vi "Load Subsystem IO Attributes.vi"(8 "error in (no error)":errorcluster, 11 "Subsystem I/O Attributes File Path":path) -> (0 "error out":errorcluster, 3 "Subsystem I/O Attributes":T1[](array[typedef]))   [LabVIEW 2024]
doc: "Load subsystem I/O attributes from the configuration file."
uses:
  Controls/Server/Subsystem IO Attributes.ctl
  Controls/Server/Subsystem IO Logging Attributes.ctl
  Controls/Server/Subsystem IO Alarm Attributes.ctl
  <vilib>/Utility/file.llb/Read Delimited Spreadsheet (string).vi
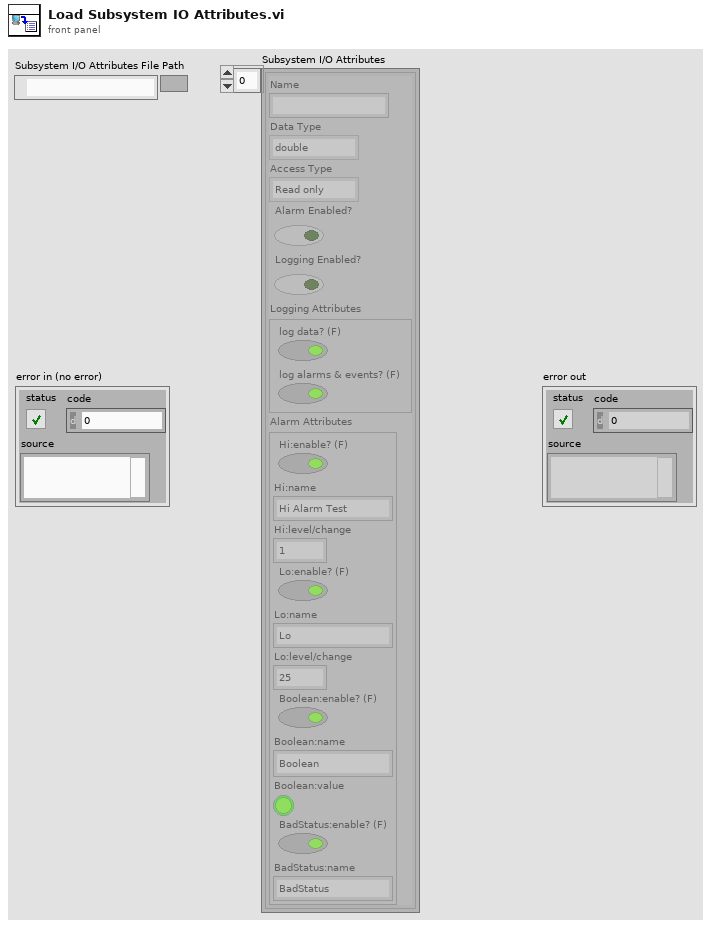
[diagram p1: front panel]
types:
  T1 = typedef "Subsystem IO Attributes.ctl" = cluster{"Name":string, "Data Type":enum32{"u32BitField", "bool", "double", "string", "int8", "uint8", "int16", "uint16", "int32", "uint32", "int64", "uint64", "single", "double waveform", "int16 waveform", "array of boolean", "array of int8", "array of uint8", "array of int16", "array of uint16", "array of int32", "array of uint32", "array of int64", "array of uint64", "array of single", "array of double", "array of double waveform", "array of int16 waveform", "array of string", "variant", "timestamp", "fixed point", "custom"}, "Access Type":enum32{"Read only", "Write only", "Read/write"}, "Alarm Enabled?":bool, "Logging Enabled?":bool, "Logging Attributes":T2, "Alarm Attributes":T3}
  T2 = typedef "Subsystem IO Logging Attributes.ctl" = cluster{"log data? (F)":bool, "log alarms & events? (F)":bool}
  T3 = typedef "Subsystem IO Alarm Attributes.ctl" = cluster{"Hi:enable? (F)":bool, "Hi:name":string, "Hi:level/change":dbl, "Lo:enable? (F)":bool, "Lo:name":string, "Lo:level/change":dbl, "Boolean:enable? (F)":bool, "Boolean:name":string, "Boolean:value":bool, "BadStatus:enable? (F)":bool, "BadStatus:name":string}
  T4 = enum32{"u32BitField", "bool", "double", "string", "int8", "uint8", "int16", "uint16", "int32", "uint32", "int64", "uint64", "single", "double waveform", "int16 waveform", "array of boolean", "array of int8", "array of uint8", "array of int16", "array of uint16", "array of int32", "array of uint32", "array of int64", "array of uint64", "array of single", "array of double", "array of double waveform", "array of int16 waveform", "array of string", "variant", "timestamp", "fixed point", "custom"}
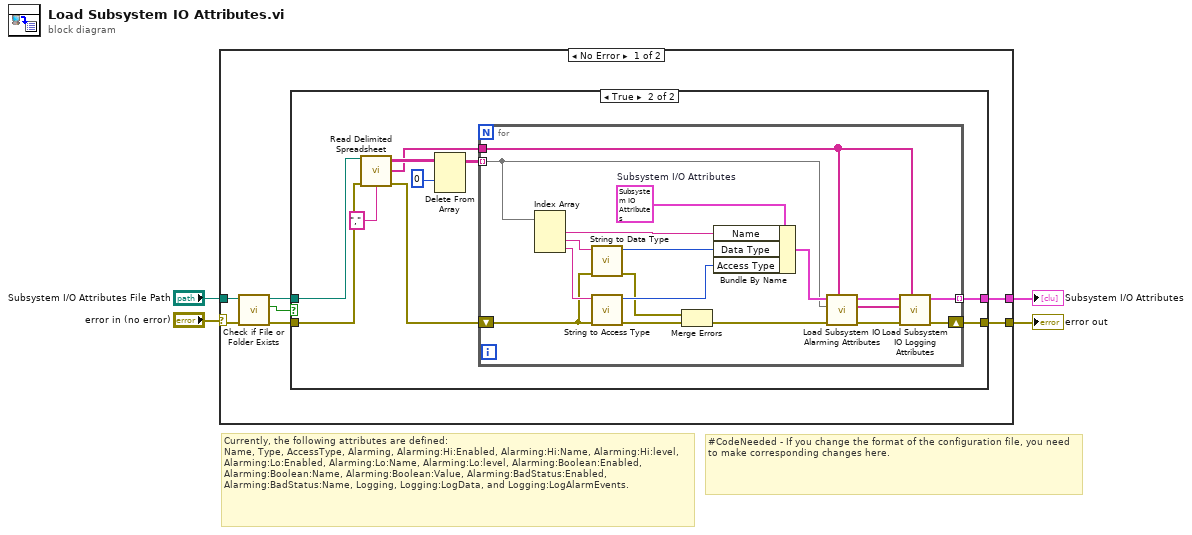
[diagram p0: block diagram]
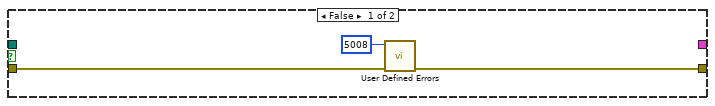
[diagram p2: hidden frame]
diagram:
  # "#CodeNeeded - If you change the format of the configuration file, you need to make corresponding changes here."
  # "Currently, the following attributes are defined:\nName, Type, AccessType, Alarming, Alarming:Hi:Enabled, Alarming:Hi:Name, Alarming:Hi:level, Alarming:Lo:Enabled, Alarming:Lo:Name, Alarming:Lo:level, Alarming:Boolean:Enabled, Alarming:Boolean:Name, Alarming:Boolean:Value, Alarming:BadStatus:Enabled, Alarming:BadStatus:Name, Logging, Logging:LogData, and Logging:LogAlarmEvents."
  n1 = case shown="No Error" "error in (no error)" {
    selector: "error in (no error)" -> [w5 w43]
    tunnel: [w11 _] -> w4
    tunnel: [w10 w43] -> w3
    tunnel: "Subsystem I/O Attributes File Path" -> [w9 _]
    frame No Error {
      n2 = call <vilib>:"Check if File or Folder Exists.vi"("error in (no error)"=w5, "path"=w9) -> ("error out"=w7:errorcluster, "file or folder exists?"=w8:bool, "dup path"=w6:path)  [unwired: 7 in]
      n3 = case shown="True" w8 {
        tunnel: [_ w20] -> w11
        tunnel: [w13 w19] -> w10
        tunnel: w7 -> [w12 w16]
        tunnel: w6 -> [_ w18]
        frame False {
          n4 = call "User Defined Errors.vi"("error in (no error)"=w12, "Error Code (0)"=5008 ("error code (0)")) -> ("error out"=w13:errorcluster)  [unwired: 9 in]
        }
        frame True {
          n5 = call-poly <vilib>:"Read Delimited Spreadsheet.vi"("file path (dialog if empty)"=w18, "error in (no error)"=w16, "delimiter (\\t)"="," ("delimiter (\\t)")) -> ("all rows"=w22:string[][], "first row"=w17:string[], "error out"=w15:errorcluster)  [unwired: 7 in, 3 out]
          n6 = Delete From Array(array=w22, index (row)=0) -> (array with subset deleted=w21:string[][])  [unwired: 2 in, 1 out]
          n7 = for {
            tunnel: w21 -> [w27] mode=indexing
            tunnel: w17 -> [w25]
            tunnel: [w29] -> w20 mode=indexing
            shift-right: [w31] -> w19
            shift-left: w15 -> [w28]
            w38 = T1 {"Name"="", "Data Type"=enum."u32BitField", "Access Type"=enum."Read only", "Alarm Enabled?"=FALSE, "Logging Enabled?"=FALSE, "Logging Attributes"={"log data? (F)"=FALSE, "log alarms & events? (F)"=FALSE}, "Alarm Attributes"={"Hi:enable? (F)"=FALSE, "Hi:name"="", "Hi:level/change"=0.0, "Lo:enable? (F)"=FALSE, "Lo:name"="", "Lo:level/change"=0.0, "Boolean:enable? (F)"=FALSE, "Boolean:name"="", "Boolean:value"=FALSE, "BadStatus:enable? (F)"=FALSE, "BadStatus:name"=""}}  # Subsystem I/O Attributes
            n8 = Index Array(array=w27) -> (element #1=w42:string, element #2=w40:string, element #3=w39:string)  [unwired: 3 in]
            n9 = call "String to Data Type.vi"("error in (no error)"=w28, "Date Type String"=w40) -> ("error out"=w36:errorcluster, "Data Type"=w41:T4)  [unwired: 8 in]
            n10 = call "String to Access Type.vi"("error in (no error)"=w28, "Access Type String"=w39) -> ("error out"=w35:errorcluster, "Access Type"=w37:enum32{"Read only", "Write only", "Read/write"})  [unwired: 8 in]
            n11 = Merge Errors(w36, w35) -> (w34:errorcluster)
            n12 = Bundle By Name(cluster=w38, "Name"=w42, "Data Type"=w41, "Access Type"=w37) -> (w33:T1)
            n13 = call "Load Subsystem IO Alarming Attributes.vi"("Headers"=w25, "error in (no error)"=w34, "Raw Configuration"=w27, "Subsystem I/O Attributes In"=w33) -> ("error out"=w32:errorcluster, "dup Raw Configuration"=w26:string[], "Subsystem I/O Attributes Out"=w30:T1)  [unwired: 5 in]
            n14 = call "Load Subsystem IO Logging Attributes.vi"("Headers"=w25, "error in (no error)"=w32, "Raw Configuration"=w26, "Subsystem I/O Attributes In"=w30) -> ("error out"=w31:errorcluster, "Subsystem I/O Item Attributes Out"=w29:T1)  [unwired: 5 in, 1 out]
          }
        }
      }
    }
    frame Error {
    }
  }
  "error out" <- w3
  "Subsystem I/O Attributes" <- w4
